vi "CreateCPUTracker.vi"(1 "height":u32=256, 2 "width":u32=256) -> (0 "return type":u64)   [LabVIEW 2011]
uses:
  CpuTrackDLL.vi
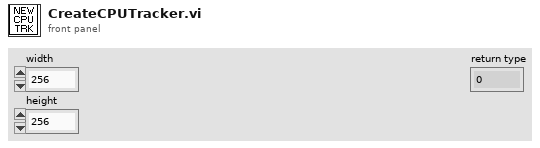
[diagram p1: front panel]
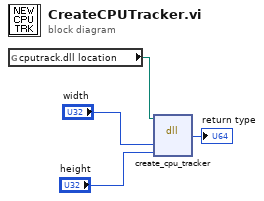
[diagram p0: block diagram]
diagram:
  n1 = global read "CpuTrackDLL.vi" "cputrack.dll location"() -> (w1:path)
  n2 = dll-call lib="D:/jcnossen1/cudaqi-tracker/Debug/cputrack.dll" fn="create_cpu_tracker"(path in=w1, "width"="width", "height"="height") -> ("return type"=→"return type":u64)  [unwired: 4 in, 2 out]
